vi "Read SG Parameters.vi"(8 "error in (no error)":errorcluster, 11 "Skyworks Spur Test in":refnum<class "Skyworks Spur Test.lvclass">) -> (0 "error out":errorcluster, 2 "SG Parameters":T1, 3 "Skyworks Spur Test out":refnum<class "Skyworks Spur Test.lvclass">)   [LabVIEW 2018, in "Skyworks Spur Test.lvlib" / "Skyworks Spur Test.lvclass"]
uses:
  Skyworks Spur Test.lvclass
  Skyworks Spur Test.lvclass/Skyworks Spur Test.ctl
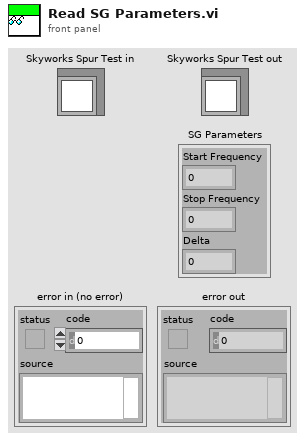
[diagram p1: front panel]
types:
  T1 = cluster{"Start Frequency":dbl, "Stop Frequency":dbl, "Delta":dbl}
  T2 = typedef "Skyworks Spur Test.lvlib/Skyworks Spur Test.lvclass/SG Parameters.ctl" = cluster{"Start Frequency":dbl, "Stop Frequency":dbl, "Delta":dbl}
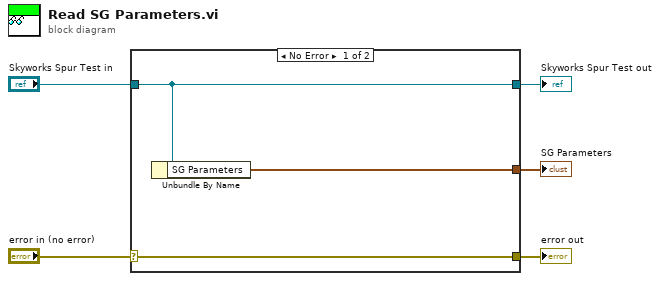
[diagram p0: block diagram]
diagram:
  n1 = case shown="No Error" "error in (no error)" {
    selector: "error in (no error)" -> [w8 w9]
    tunnel: [w8 w9] -> w4
    tunnel: [w7 w10] -> w2
    tunnel: "Skyworks Spur Test in" -> [w7 w10]
    tunnel: [w6 _] -> w1
    frame No Error {
      n2 = Unbundle By Name(w7) -> ("SG Parameters"=w6:T2)
    }
    frame Error {
    }
  }
  "error out" <- w4
  "Skyworks Spur Test out" <- w2
  "SG Parameters" <- w1
